vi "0x2 RIO-OCU command receive.vi"(11 "Manual Override Reader In":refnum<class "NetworkStreamReader.lvclass">) -> (3 "Manual Override Reader Out":refnum<class "NetworkStreamReader.lvclass">)   [LabVIEW 2011]
doc: "Gets commands from the OCU and sends them out to the rest of the code on the RIO using the globals."
uses:
  2-Think/2 Typedefs/rudder angle.ctl
  2-Think/2 Typedefs/sail setpt.ctl
  2-Think/2 Typedefs/setpoints to boat.ctl
  0x2 Typedefs/manual override.ctl
  0x2 Typedefs/Current Waypoint.ctl
  2-Think/2 Globals/2 Global.vi
  0x2 Typedefs/ocuCommands.ctl
  0x2 Typedefs/ocuMessage.ctl
  0x2 Classes/NetworkStreams/Reader/NetworkStreamReader.lvclass
  2-Think/2 Classes/MissionQueue/MissionQueue.lvclass
  2-Think/2 Classes/Missions/GenericMission/GenericMission.lvclass
  2-Think/2 Globals/2 TuningConstants.vi
  2-Think/2 Typedefs/UTM Circle.ctl
  2-Think/2 Typedefs/Goodness Weightings.ctl
  2-Think/2 Typedefs/PI Constants.ctl
  2-Think/2 Typedefs/Apparent Wind Mode.ctl
  0x2 Typedefs/Control values.ctl
  2-Think/2 Classes/Logger/Logger.lvclass
  2-Think/2 Globals/2 Message Logger.vi
  0x2 Typedefs/Sail Setting Tuning.ctl
panel:
  out "Latest OCU Command":T1
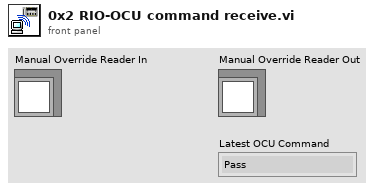
[diagram p1: front panel]
types:
  T1 = typedef "ocuCommands.ctl" = enum16{"Pass", "Send override", "Set waypoint number", "Stop", "Add Mission", "Reset Missions/Waypts", "Edit Control Values", "Add Global No-Sail", "Log Message"}
  T2 = typedef "manual override.ctl" = cluster{"Override Active Rudder":bool, "Setpoints":T3, "Override Active Sail":bool}
  T3 = typedef "setpoints to boat.ctl" = cluster{"Sail Position":T4, "Rudder Angle":T5}
  T4 = typedef "sail setpt.ctl" = dbl
  T5 = typedef "rudder angle.ctl" = dbl
  T6 = typedef "ocuMessage.ctl" = cluster{"OCU Command":T1, "Data":variant}
  T7 = typedef "UTM Circle.ctl" = cluster{"UTM Zone":dbl, "Hemisphere":enum16{"North", "South"}, "East":dbl, "North":dbl, "Radius":dbl}
  T8 = typedef "Current Waypoint.ctl" = i32
  T9 = typedef "Control values.ctl" = cluster{"Goodness Weightings":T10, "PI Constants":T11, "No Sail Zone\nTuning Quotient":dbl, "Heading Change Wind Adjustment":dbl, "Waypoint Tuning Quotient":dbl, "Apparent Wind Mode":T12, "Let Sail Out on Windcross":bool, "Shift Goal for currents":bool, "Round Buoy Safety":dbl, "Sail Setting Options":T13, "Defilter Wind Data":bool, "Irons Range":dbl, "Force tack attempt?":bool, "Minimum\ntack try\ntime?":dbl}
  T10 = typedef "Goodness Weightings.ctl" = cluster{"Target Importance":dbl, "No Sail Importance":dbl, "Change Importance":dbl, "Pure Waypoint \nImportance":dbl, "Pure Wind \nImportance":dbl}
  T11 = typedef "PI Constants.ctl" = cluster{"Proportional Gain":dbl, "Integral Time":dbl, "Derivative Time":dbl}
  T12 = typedef "Apparent Wind Mode.ctl" = cluster{"Desired Apparent\nWind Direction":dbl, "On":bool}
  T13 = typedef "Sail Setting Tuning.ctl" = cluster{"Linear\nMode":bool, "Sails Full In Point":dbl, "Sails Full Out Point":dbl}
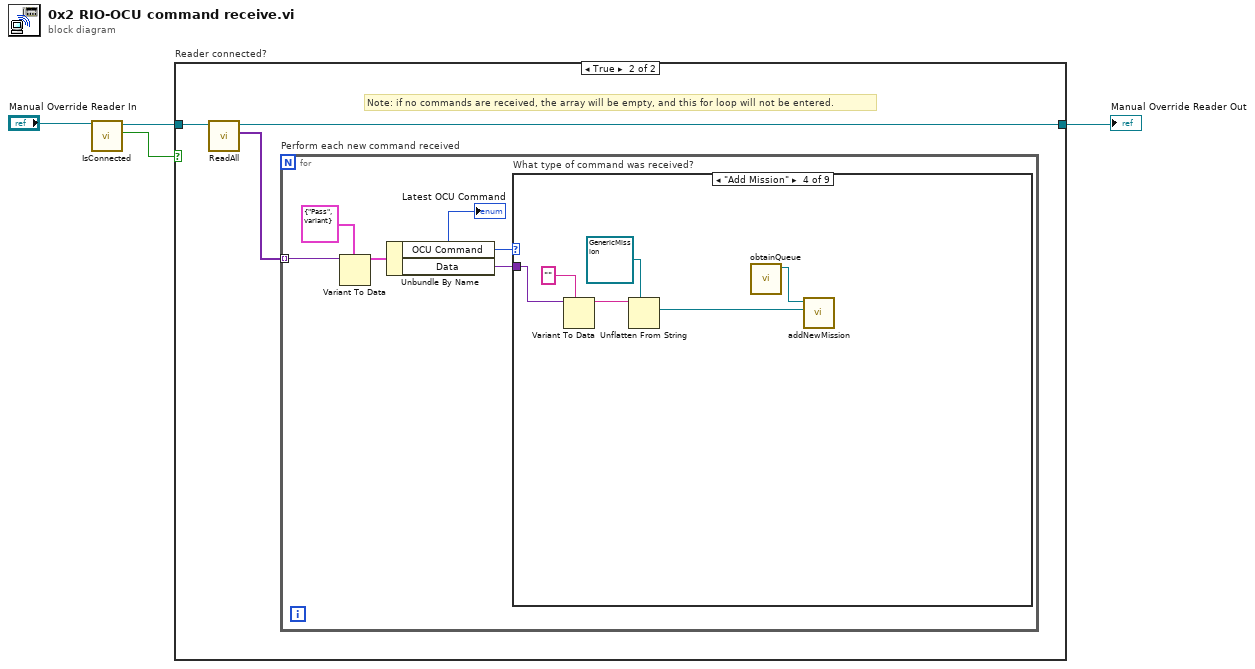
[diagram p0: block diagram]
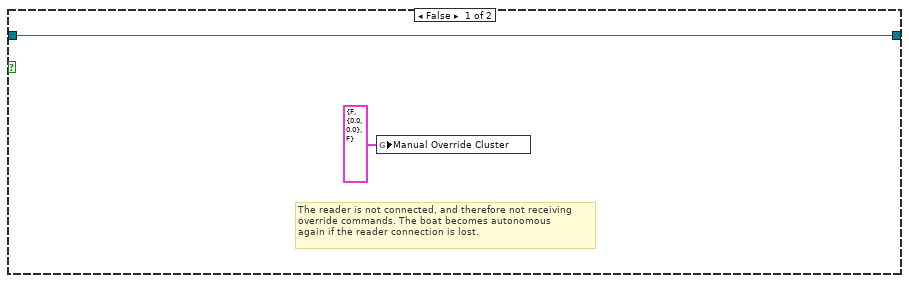
[diagram p2: hidden frame]
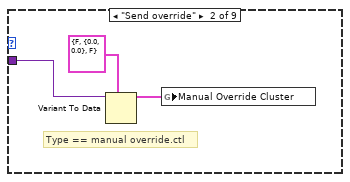
[diagram p4: hidden frame]
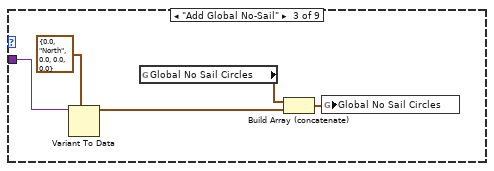
[diagram p5: hidden frame]
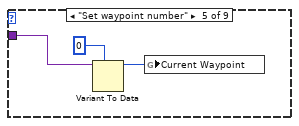
[diagram p6: hidden frame]
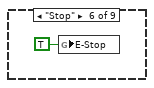
[diagram p7: hidden frame]
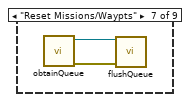
[diagram p8: hidden frame]
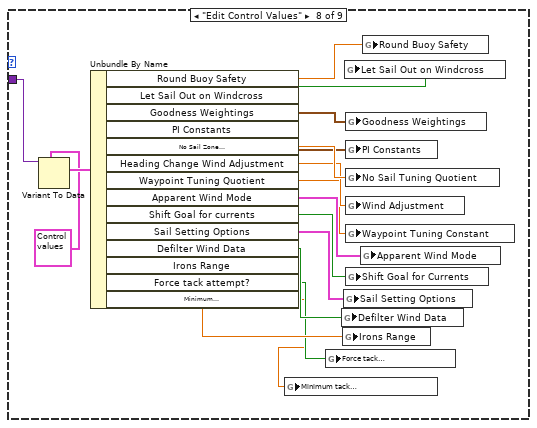
[diagram p9: hidden frame]
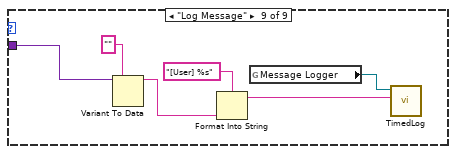
[diagram p10: hidden frame]
diagram:
  n1 = call "IsConnected.vi"("NetworkStreamReader in"="Manual Override Reader In") -> ("Connected?"=w3:bool, "NetworkStreamReader out"=w2:refnum<class "NetworkStreamReader.lvclass">)  [unwired: 8 in, 1 out]
  n2 = case "Reader connected?" shown="True" w3 {
    tunnel: w2 -> [w5 w8]
    tunnel: [w5 w7] -> w1
    frame False {
      # "The reader is not connected, and therefore not receiving\noverride commands. The boat becomes autonomous \nagain if the reader connection is lost."
      n3 = global write "2 Global.vi" "Manual Override Cluster"(T2 {"Override Active Rudder"=FALSE, "Setpoints"={"Sail Position"=0.0, "Rudder Angle"=0.0}, "Override Active Sail"=FALSE} ("Manual Override Cluster")) -> ()
    }
    frame True {
      # "Note: if no commands are received, the array will be empty, and this for loop will not be entered."
      n4 = call "ReadAll.vi"("NetworkStreamReader in"=w8) -> ("elements"=w9:variant[], "NetworkStreamReader out"=w7:refnum<class "NetworkStreamReader.lvclass">)  [unwired: 6 in, 3 out]
      n5 = for "Perform each new command received" {
        tunnel: w9 -> [w10] mode=indexing
        n6 = Variant To Data(type=T6 {"OCU Command"=enum."Pass", "Data"=variant} ("OCU Message"), Variant=w10) -> (data=w13:T6)  [unwired: 1 in, 1 out]
        n7 = Unbundle By Name(w13) -> ("OCU Command"=w12:T1, "Data"=w11:variant)
        "Latest OCU Command" <- w12
        n8 = case "What type of command was received?" shown="\"Add Mission\"" w12 {
          tunnel: w11 -> [_ w16 w22 w26 w31 _ _ w51 w56]
          frame "Pass", Default {
          }
          frame "Send override" {
            # "Type == manual override.ctl"
            n9 = Variant To Data(type=T2 {"Override Active Rudder"=FALSE, "Setpoints"={"Sail Position"=0.0, "Rudder Angle"=0.0}, "Override Active Sail"=FALSE} ("Manual Override Cluster"), Variant=w16) -> (data=w15:T2)  [unwired: 1 in, 1 out]
            n10 = global write "2 Global.vi" "Manual Override Cluster"(w15) -> ()
          }
          frame "Add Global No-Sail" {
            n11 = Variant To Data(type=T7 {"UTM Zone"=0.0, "Hemisphere"=enum."North", "East"=0.0, "North"=0.0, "Radius"=0.0} ("UTM Location"), Variant=w22) -> (data=w18:T7)  [unwired: 1 in, 1 out]
            n12 = global read "2 Global.vi" "Global No Sail Circles"() -> (w21:T7[])
            n13 = Build Array (concatenate)(w21, w18) -> (w20:T7[])
            n14 = global write "2 Global.vi" "Global No Sail Circles"(w20) -> ()
          }
          frame "Add Mission" {
            n15 = Variant To Data(type="", Variant=w26) -> (data=w27:string)  [unwired: 1 in, 1 out]
            n16 = Unflatten From String(type=refnum<class "GenericMission.lvclass"> refnum ("GenericMission.lvclass"), binary string=w27) -> (value=w23:refnum<class "GenericMission.lvclass">)  [unwired: 3 in, 2 out]
            n17 = call "obtainQueue.vi"() -> ("MissionQueue.lvclass"=w24:refnum<class "MissionQueue.lvclass">)  [unwired: 10 in, 1 out]
            n18 = call "addNewMission.vi"("GenericMission.lvclass"=w23, "MissionQueue in"=w24) -> ()  [unwired: 8 in, 2 out]
          }
          frame "Set waypoint number" {
            n19 = Variant To Data(type=T8 0 ("Current Waypoint"), Variant=w31) -> (data=w29:T8)  [unwired: 1 in, 1 out]
            n20 = global write "2 Global.vi" "Current Waypoint"(w29) -> ()
          }
          frame "Stop" {
            n21 = global write "2 Global.vi" "E-Stop"(TRUE ("E-Stop")) -> ()
          }
          frame "Reset Missions/Waypts" {
            n22 = call "obtainQueue.vi"() -> ("Error Out"=w33:errorcluster, "MissionQueue.lvclass"=w34:refnum<class "MissionQueue.lvclass">)  [unwired: 10 in]
            n23 = call "flushQueue.vi"("error in (no error)"=w33, "MissionQueue in"=w34) -> ()  [unwired: 7 in, 3 out]
          }
          frame "Edit Control Values" {
            n24 = Variant To Data(type=T9 {"Goodness Weightings"={"Target Importance"=0.0, "No Sail Importance"=0.0, "Change Importance"=0.0, "Pure Waypoint \nImportance"=0.0, "Pure Wind \nImportance"=0.0}, "PI Constants"={"Proportional Gain"=0.0, "Integral Time"=0.0, "Derivative Time"=0.0}, "No Sail Zone\nTuning Quotient"=0.0, "Heading Change Wind Adjustment"=0.0, "Waypoint Tuning Quotient"=0.0, "Apparent Wind Mode"={"Desired Apparent\nWind Direction"=0.0, "On"=FALSE}, "Let Sail Out on Windcross"=FALSE, "Shift Goal for currents"=FALSE, "Round Buoy Safety"=0.0, "Sail Setting Options"={"Linear\nMode"=FALSE, "Sails Full In Point"=0.0, "Sails Full Out Point"=0.0}, "Defilter Wind Data"=FALSE, "Irons Range"=0.0, "Force tack attempt?"=FALSE, "Minimum\ntack try\ntime?"=0.0}, Variant=w51) -> (data=w50:T9)  [unwired: 1 in, 1 out]
            n25 = Unbundle By Name(w50) -> ("Round Buoy Safety"=w40:dbl, "Let Sail Out on Windcross"=w42:bool, "Goodness Weightings"=w48:T10, "PI Constants"=w47:T11, "No Sail Zone\nTuning Quotient"=w49:dbl, "Heading Change Wind Adjustment"=w46:dbl, "Waypoint Tuning Quotient"=w45:dbl, "Apparent Wind Mode"=w43:T12, "Shift Goal for currents"=w41:bool, "Sail Setting Options"=w39:T13, "Defilter Wind Data"=w38:bool, "Irons Range"=w37:dbl, "Force tack attempt?"=w36:bool, "Minimum\ntack try\ntime?"=w35:dbl)
            n26 = global write "2 TuningConstants.vi" "Minimum tack\ntry time?"(w35) -> ()
            n27 = global write "2 TuningConstants.vi" "Force tack\nattempt?"(w36) -> ()
            n28 = global write "2 Global.vi" "Defilter Wind Data"(w38) -> ()
            n29 = global write "2 TuningConstants.vi" "Irons Range"(w37) -> ()
            n30 = global write "2 TuningConstants.vi" "Sail Setting Options"(w39) -> ()
            n31 = global write "2 Global.vi" "Let Sail Out on Windcross"(w42) -> ()
            n32 = global write "2 TuningConstants.vi" "Goodness Weightings"(w48) -> ()
            n33 = global write "2 TuningConstants.vi" "PI Constants"(w47) -> ()
            n34 = global write "2 TuningConstants.vi" "No Sail Tuning Quotient"(w49) -> ()
            n35 = global write "2 TuningConstants.vi" "Wind Adjustment"(w46) -> ()
            n36 = global write "2 TuningConstants.vi" "Waypoint Tuning Constant"(w45) -> ()
            n37 = global write "2 Global.vi" "Shift Goal for Currents"(w41) -> ()
            n38 = global write "2 TuningConstants.vi" "Apparent Wind Mode"(w43) -> ()
            n39 = global write "2 Global.vi" "Round Buoy Safety"(w40) -> ()
          }
          frame "Log Message" {
            n40 = Variant To Data(type="" ("Message"), Variant=w56) -> (data=w53:string)  [unwired: 1 in, 1 out]
            n41 = Format Into String(format string="[User] %s", w53) -> (resulting string=w52:string)  [unwired: 2 in, 1 out]
            n42 = global read "2 Message Logger.vi" "Message Logger"() -> (w55:refnum<class "Logger.lvclass">)
            n43 = call "TimedLog.vi"("Message"=w52, "Logger in"=w55) -> ()  [unwired: 7 in, 3 out]
          }
        }
      }
    }
  }
  "Manual Override Reader Out" <- w1
